vi "Delay Boolean.vi"(1 "Mode":T1(ring), 3 "Invert":bool, 5 "input":bool, 9 "Delay":i32) -> (6 "Output":bool, 8 "Debounced":bool, 10 "History":bool[](array[boolean]))   [LabVIEW 2016]
doc: "Every milisecond this VI inserts the value of the input terminal into an array at an index equal to delay pushing every other value in the array one index toward zero. The output terminal is equal to the zero index of the array. The array can be retrived from the history terminal and the average of the array can be retrived from the debounced terminal.\n\nThe mode terminal sets the mode of the delay. when the mode is set to falling the VI reinitializes the entire array as true when the button is pressed. In falling mode it reintitializes it as false when the button is released. Neither mode will not reinitalize when the input changes. Instant mode will remove the milisecond wait and complete all of the tasks once per cycle.\n\nWhen the Value of the delay terminal is changed the array is reinitialized as false.\n\nWhen the boolean polymorphic subVI recives true on the invert terminal it inverts it's input and all array initializations/reinitializations.\n\nWhen the doubble or integer polymorphic subVI is set to falling mode it sends the input directly to the output until it is set to zero. when set to zero it will send the last non zero value for delay ms. Rising mode does the opposite. \n\nCreated by Team 4130 for use in the 2016-2017 FRC season"
uses:
  <vilib>/Analysis/baseanly.llb/Mean (DBL).vi
  <vilib>/Analysis/NI_AALBase.lvlib
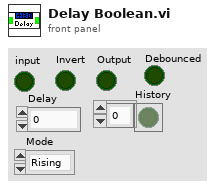
[diagram p1: front panel]
types:
  T1 = enum16{"Rising", "Falling", "Neither", "Instant"}
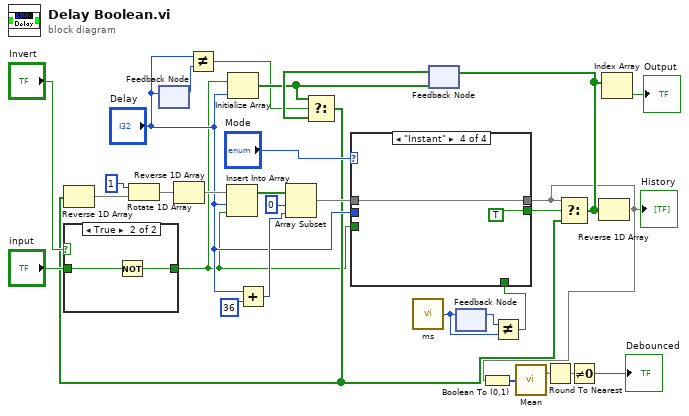
[diagram p0: block diagram]
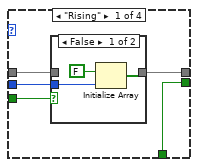
[diagram p3: hidden frame]
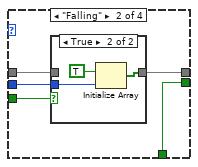
[diagram p5: hidden frame]
diagram:
  n1 = case shown="True" "Invert" {
    tunnel: [w31 w32] -> w4
    tunnel: "input" -> [w31 w33]
    frame False {
    }
    frame True {
      n2 = Not(x=w33) -> (.not. x?=w32:bool)
    }
  }
  n3 = feedback #1() -> (w9:i32)  [unwired: 1 in]
  n4 = feedback-in #1("Delay") -> ()
  n5 = Not Equal?(x="Delay", y=w9) -> (x != y?=w5:bool)
  n6 = Initialize Array(w4, "Delay") -> (w6:bool[])
  n7 = Add(x="Delay", y=36) -> (x+y=w17:i32)
  n8 = call "ms.vi"() -> ("millisecond"=w29:u32)  [unwired: 1 in]
  n9 = feedback #2(w6) -> (w7:bool[])
  n10 = Select(t=w6, s=w5, f=w7) -> (s? t:f=w8:bool[])
  n11 = Reverse 1D Array(array=w8) -> (reversed array=w26:bool[])
  n12 = Rotate 1D Array(1:w26, 2:1 ("n")) -> (0:w28:bool[])
  n13 = Reverse 1D Array(array=w28) -> (reversed array=w25:bool[])
  n14 = Insert Into Array(array=w25, index="Delay", new element=w4) -> (w19:bool[])
  n15 = Array Subset(array=w19, index=0, length=w17) -> (w18:bool[])
  n16 = feedback #3() -> (w30:u32)  [unwired: 1 in]
  n17 = feedback-in #3(w29) -> ()
  n18 = Not Equal?(x=w30, y=w29) -> (x != y?=w3:bool)
  n19 = case shown="\"Instant\"" "Mode" {
    tunnel: w18 -> [w36 w46 w53 w55]
    tunnel: [w37 w45 w53 w55] -> w1
    tunnel: w4 -> [w38 w47 _ _]
    tunnel: "Delay" -> [w35 w44 _ _]
    tunnel: w3 -> [w34 w43 w52 _]
    tunnel: [w34 w43 w52 TRUE] -> w2
    frame "Rising" {
      n20 = case shown="False" w38 {
        tunnel: [w40 w42] -> w37
        tunnel: w36 -> [_ w42]
        tunnel: w35 -> [w41 _]
        frame False {
          n21 = Initialize Array(FALSE, w41) -> (w40:bool[])
        }
        frame True {
        }
      }
    }
    frame "Falling" {
      n22 = case shown="True" w47 {
        tunnel: [w48 w50] -> w45
        tunnel: w46 -> [w48 _]
        tunnel: w44 -> [_ w51]
        frame False {
        }
        frame True {
          n23 = Initialize Array(TRUE, w51) -> (w50:bool[])
        }
      }
    }
    frame "Neither", Default {
    }
    frame "Instant" {
    }
  }
  "History" <- w1
  n24 = Boolean To (0,1)(Boolean=w1) -> (0, 1=w14:i16[])
  n25 = call-poly <vilib>:"Mean.vi"("X"=w14) -> ("mean"=w13:dbl)  [unwired: 1 out]
  n26 = Round To Nearest(number=w13) -> (nearest integer value=w12:dbl)
  n27 = Select(t=w1, s=w2, f=w8) -> (s? t:f=w23:bool[])
  n28 = feedback-in #2(w23) -> ()
  n29 = Not Equal To 0?(x=w12) -> (x != 0?=→"Debounced":bool)
  n30 = Reverse 1D Array(array=w23) -> ()  [unwired: 1 out]
  n31 = Index Array(array=w23) -> (element=→"Output":bool)  [unwired: 1 in]
